vi "Set_4G_RLC_Timer_Poll_Retransmit.vi"(8 "error in (no error)":errorcluster, 10 "value":i32=80 min=0 max=500 step=5, 11 "Base Station":T1) -> (0 "error out":errorcluster, 3 "Output String":string)   [LabVIEW 2021]
uses:
  Controls/Base_Station_Emulator.ctl
  Controls/TCP_FGV.ctl
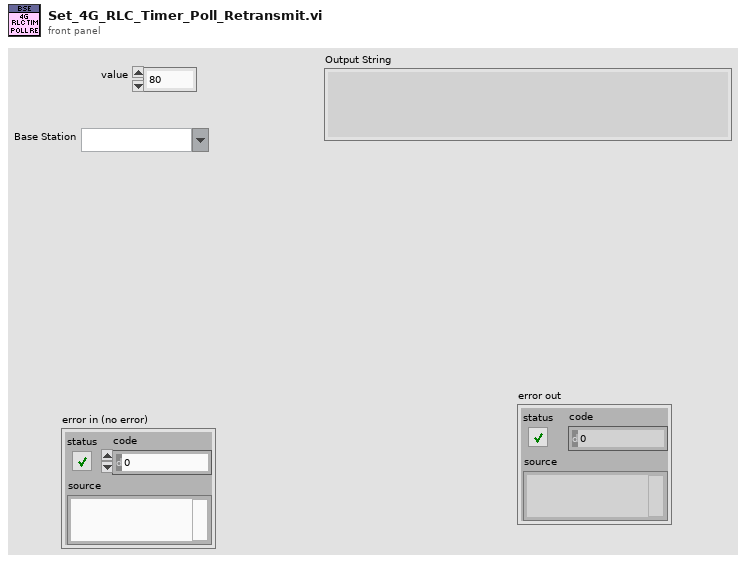
[diagram p1: front panel]
types:
  T1 = typedef "Base_Station_Emulator.ctl" = string
  T2 = typedef "TCP_FGV.ctl" = enum16{"Open", "Read", "Write", "Close"}
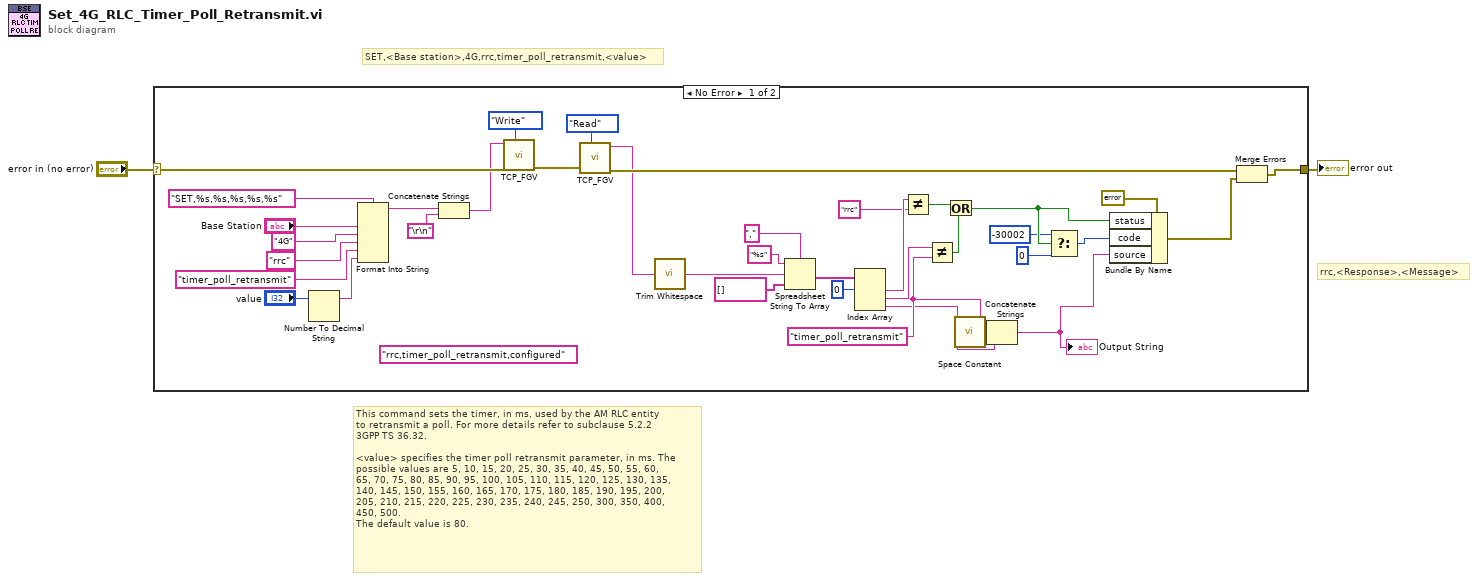
[diagram p0: block diagram]
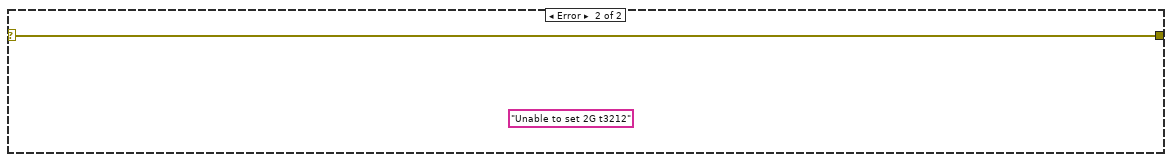
[diagram p2: hidden frame]
diagram:
  # "This command sets the timer, in ms, used by the AM RLC entity \nto retransmit a poll. For more details refer to subclause 5.2.2 \n3GPP TS 36.32. \n\n<value> specifies the timer poll retransmit parameter, in ms. The \npossible values are 5, 10, 15, 20, 25, 30, 35, 40, 45, 50, 55, 60, \n65, 70, 75, 80, 85, 90, 95, 100, 105, 110, 115, 120, 125, 130, 135, \n140, 145, 150, 155, 160, 165, 170, 175, 180, 185, 190, 195, 200, \n205, 210, 215, 220, 225, 230, 235, 240, 245, 250, 300, 350, 400, \n450, 500.\nThe default value is 80."
  # "SET,<Base station>,4G,rrc,timer_poll_retransmit,<value>"
  # "rrc,<Response>,<Message>"
  n1 = case shown="No Error" "error in (no error)" {
    selector: "error in (no error)" -> [w37 w41]
    tunnel: [w14 w41] -> w1
    frame No Error {
      (unwired) "rrc,timer_poll_retransmit,configured" ("format string")
      w12 = "timer_poll_retransmit"
      n2 = Number To Decimal String(number="value") -> (decimal integer string=w7:string)  [unwired: 1 in]
      n3 = Format Into String(format string="SET,%s,%s,%s,%s,%s", "Base Station", "4G", "rrc", "timer_poll_retransmit", w7) -> (resulting string=w5:string)  [unwired: 2 in, 1 out]
      n4 = Concatenate Strings(w5, "\r\n") -> (w4:string)
      n5 = call "TCP_FGV.vi"("Command"=w4, "error in (no error)"=w37, "Operation"=TCP_FGV."Write") -> ("error out"=w15:errorcluster)  [unwired: 6 in, 1 out]
      n6 = call "TCP_FGV.vi"("error in (no error)"=w15, "Operation"=TCP_FGV."Read") -> ("Data Out"=w3:string, "error out"=w17:errorcluster)  [unwired: 7 in]
      n7 = call <vilib>:"Trim Whitespace.vi"("string"=w3) -> ("trimmed string"=w31:string)  [unwired: 1 in]
      n8 = Spreadsheet String To Array(delimiter (Tab)=",", format string="%s", spreadsheet string=w31, array type (2D Dbl)=string[] []) -> (array=w27:string[])
      n9 = Index Array(array=w27, index #1=0 ("index")) -> (element #1=w28:string, element #2=w18:string, element #3=w11:string)  [unwired: 2 in]
      n10 = Not Equal?(x=w28, y="rrc" ("format string")) -> (x != y?=w29:bool)
      n11 = Not Equal?(x=w18, y=w12) -> (x != y?=w30:bool)
      n12 = Or(x=w29, y=w30) -> (x .or. y?=w32:bool)
      n13 = call <vilib>:"Space Constant.vi"() -> ("String"=w13:string)
      n14 = Concatenate Strings(w12, w13, w11) -> (w10:string)
      "Output String" <- w10
      n15 = Select(t=-30002 ("code"), s=w32, f=0 ("code")) -> (s? t:f=w33:i32)
      n16 = Bundle By Name(cluster=errorcluster {"status"=FALSE, "code"=0, "source"=""} ("error constant"), "status"=w32, "code"=w33, "source"=w10) -> (w16:errorcluster)
      n17 = Merge Errors(w17, w16) -> (w14:errorcluster)
    }
    frame Error {
      (unwired) "Unable to set 2G t3212" ("source")
    }
  }
  "error out" <- w1
